vi "Get Routes.vi"(8 "error in (no error)":errorcluster, 11 "MuxAPI in":refnum<class "MuxAPI.lvclass">) -> (0 "error out":errorcluster, 2 "Routes":cluster{"Mux Route":i32[]}[](array[cluster]), 3 "MuxAPI out":refnum<class "MuxAPI.lvclass">)   [LabVIEW 2022 SP3, in "VideoMux.lvlib" / "MuxAPI.lvclass"]
uses:
  MuxAPI.lvclass
  MuxAPI.lvclass/MuxAPI.ctl
  <vilib>/IlluminatedG/IG Promises/Promises/Promise/Promise.lvclass
  MuxRoute Value/MuxRoute Value.lvclass
  <vilib>/IlluminatedG/IG Promises/Promises/Future/Future.lvclass
  C:/Program Files (x86)/National Instruments/LabVIEW 2022/vi.lib/IlluminatedG/IG Promises/Promises/Value/Value.lvclass
  C:/dev/illuminatedg/TouchControl/VideoMux/MuxRoute Value/MuxRoute Value.lvclass
  MuxActor Messages/Get Routes Msg/Get Routes Msg.lvclass
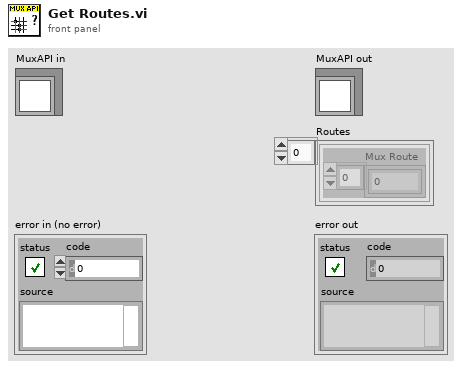
[diagram p1: front panel]
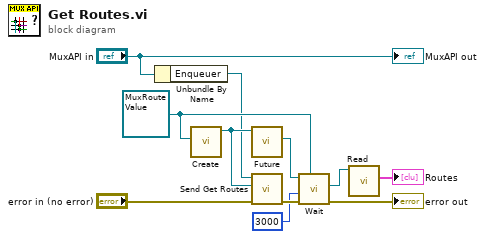
[diagram p0: block diagram]
diagram:
  w8 = refnum<class "MuxRoute Value.lvclass"> refnum ("VideoMux.lvlib:MuxRoute Value.lvclass")
  n1 = Unbundle By Name("MuxAPI in") -> ("Enqueuer"=w1:refnum<class "Message Enqueuer.lvclass">)
  n2 = call <vilib>:"Create.vi"("Result Type"=w8) -> ("Promise"=w9:refnum<class "Promise.lvclass">)  [unwired: 9 in, 1 out]
  n3 = call <vilib>:"Future.vi"("Promise in"=w9) -> ("Future"=w3:refnum<class "Future.lvclass">)  [unwired: 9 in, 1 out]
  n4 = call "Send Get Routes.vi"("error in (no error)"="error in (no error)", "Promise in"=w9, "Message Enqueuer"=w1) -> ("error out"=w7:errorcluster)  [unwired: 7 in, 1 out]
  n5 = call <vilib>:"Wait.vi"("Result Type"=w8, "error in (no error)"=w7, "Timeout mS (-1)"=3000, "Future in"=w3) -> ("error out"=→"error out":errorcluster, "Result"=w5:refnum<class "MuxRoute Value.lvclass">)  [unwired: 6 in]
  n6 = call "Read.vi"("MuxRoute Value in"=w5) -> ("Muxes"=→"Routes":cluster{"Mux Route":i32[]}[])  [unwired: 10 in]
  "MuxAPI out" <- "MuxAPI in"
